vi "VISAs2NMLAddresses.vi"(1 "VISA Resource Names":refnum<visa-resource-name>[](array[refnum])) -> (0 "NML Addresses":string[](array[string]))   [LabVIEW 2019]
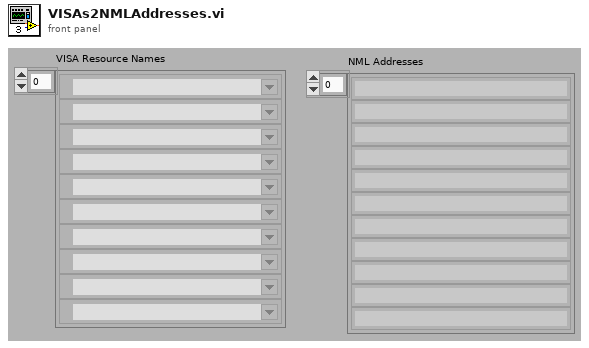
[diagram p1: front panel]
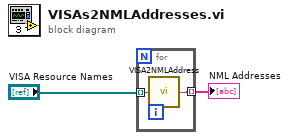
[diagram p0: block diagram]
diagram:
  n1 = for {
    tunnel: [w4] -> w2 mode=indexing
    tunnel: "VISA Resource Names" -> [w3] mode=indexing
    n2 = call "VISA2NMLAddress.vi"("VISA resource name"=w3) -> ("NML Address"=w4:string)
  }
  "NML Addresses" <- w2
